vi "destroyInternal.vi"(8 "error in (no error)":errorcluster, 11 "UserEvents in":refnum<class "UserEvents.lvclass">) -> (0 "error out":errorcluster, 3 "UserEvents out":refnum<class "UserEvents.lvclass">)   [LabVIEW 2016, in "UserEvents.lvclass"]
uses:
  UserEvents.lvclass
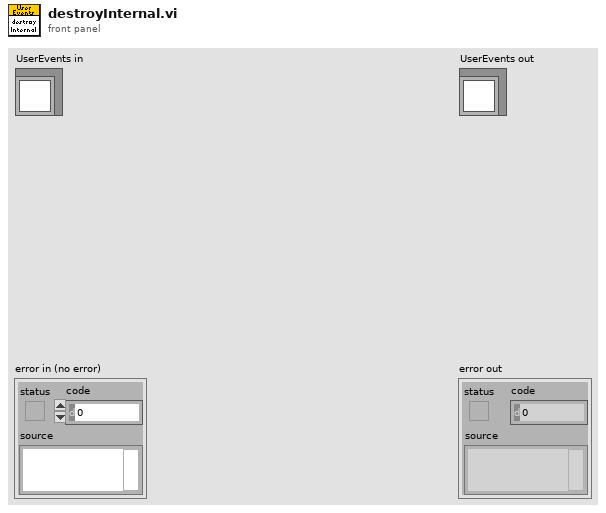
[diagram p1: front panel]
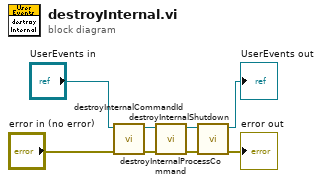
[diagram p0: block diagram]
diagram:
  n1 = call "destroyInternalCommandId.vi"("error in (no error)"="error in (no error)", "UserEvents in"="UserEvents in") -> ("error out"=w3:errorcluster, "UserEvents out"=w7:refnum<class "UserEvents.lvclass">)  [unwired: 8 in]
  n2 = call "destroyInternalProcessCommand.vi"("error in (no error)"=w3, "UserEvents in"=w7) -> ("error out"=w2:errorcluster, "UserEvents out"=w6:refnum<class "UserEvents.lvclass">)  [unwired: 8 in]
  n3 = call "destroyInternalShutdown.vi"("error in (no error)"=w2, "UserEvents in"=w6) -> ("error out"=→"error out":errorcluster, "UserEvents out"=→"UserEvents out":refnum<class "UserEvents.lvclass">)  [unwired: 8 in]
